vi "Ch_data_pattern_4_save (SubVI).vi"(0 "1":dbl, 1 "2":dbl, 2 "3":dbl, 3 "4":dbl, 14 "file":refnum<file>, 15 "Activate!":bool) -> (27 "error out":errorcluster)   [LabVIEW 2015]
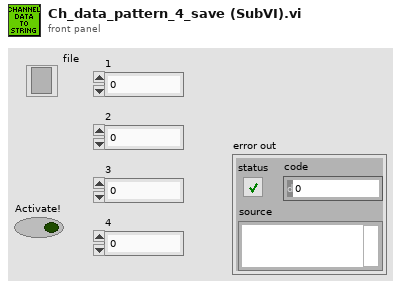
[diagram p1: front panel]
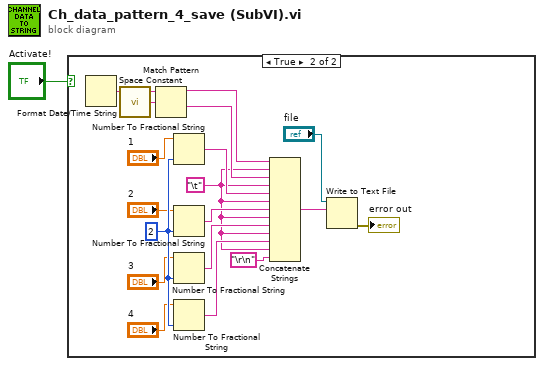
[diagram p0: block diagram]
diagram:
  n1 = case shown="True" "Activate!" {
    frame False {
    }
    frame True {
      w19 = i16 2 ("precision (6)")
      w3 = "\t"
      n2 = Format Date/Time String() -> (date/time string=w10:string)  [unwired: 3 out]
      n3 = call <vilib>:"Space Constant.vi"() -> ("String"=w11:string)
      n4 = Match Pattern(string=w10, regular expression=w11) -> (before substring=w12:string, after substring=w13:string)  [unwired: 3 out]
      n5 = Number To Fractional String(number="1", precision (6)=w19) -> (F-format string=w15:string)  [unwired: 2 out]
      n6 = Number To Fractional String(number="2", precision (6)=w19) -> (F-format string=w16:string)  [unwired: 2 out]
      n7 = Number To Fractional String(number="3", precision (6)=w19) -> (F-format string=w17:string)  [unwired: 2 out]
      n8 = Number To Fractional String(number="4", precision (6)=w19) -> (F-format string=w18:string)  [unwired: 2 out]
      n9 = Concatenate Strings(w12, w3, w13, w3, w15, w3, w16, w3, w17, w3, w18, w3, "\r\n") -> (w6:string)
      n10 = Write to Text File(file (use dialog)="file", text=w6) -> (error out=→"error out":errorcluster)  [unwired: 1 in, 3 out]
    }
  }
